vi "Read configuration.vi"(7 "force loading?":bool=TRUE, 8 "error in (no error)":errorcluster, 11 "RSA in":refnum<class "RSA.lvclass">) -> (0 "error out":errorcluster, 3 "RSA out":refnum<class "RSA.lvclass">)   [LabVIEW 2012, in "RSA.lvclass"]
doc: "Reads the XML-based configuration file and populates the configuration cluster accordingly. Configuration file name is <component ID>.xml."
uses:
  RSA.lvclass
  <vilib>/Distrio/Murmex/Murmex/Murmex.lvclass
  RSA.lvclass/RSA.ctl
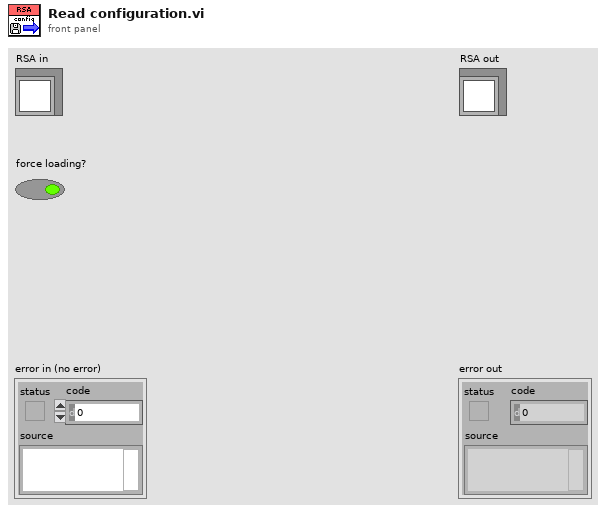
[diagram p1: front panel]
types:
  T1 = typedef "RSA.lvclass/configurationcluster.ctl" = cluster{"initialised array":dbl[]}
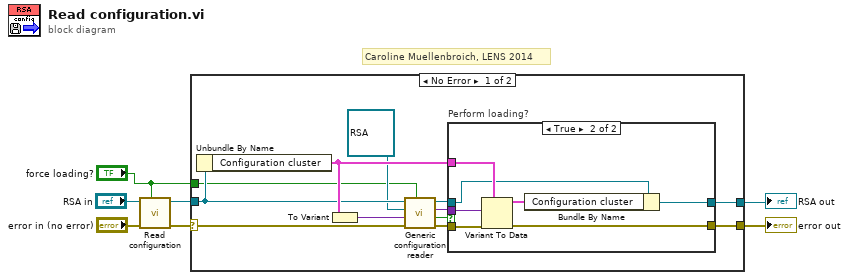
[diagram p0: block diagram]
diagram:
  # "Caroline Muellenbroich, LENS 2014"
  n1 = call-parent "Read configuration.vi"("force loading?"="force loading?", "error in (no error)"="error in (no error)", "Murmex in"="RSA in") -> ("error out"=w5:errorcluster, "Murmex out"=w4:refnum<class "RSA.lvclass">)  [unwired: 7 in]
  n2 = case shown="No Error" w5 {
    selector: w5 -> [w16 w29]
    tunnel: w4 -> [w11 w30]
    tunnel: [w18 w30] -> w3
    tunnel: [w17 w29] -> w2
    tunnel: "force loading?" -> [w8 _]
    frame No Error {
      n3 = Unbundle By Name(w11) -> ("Configuration cluster"=w19:T1)
      n4 = To Variant(anything=w19) -> (Variant=w9:variant)
      n5 = call <vilib>:"Generic configuration reader.vi"("force loading?"=w8, "error in (no error)"=w16, "configuration cluster variant"=w9, "inheritance level"=refnum<class "RSA.lvclass"> refnum ("RSA"), "Murmex in"=w11) -> ("error out"=w15:errorcluster, "loaded?"=w14:bool, "configuration data (variant)"=w13:variant, "Murmex out"=w12:refnum<class "RSA.lvclass">)  [unwired: 3 in]
      n6 = case "Perform loading?" shown="True" w14 {
        tunnel: w19 -> [_ w28]
        tunnel: [w21 w26] -> w17
        tunnel: [w20 w25] -> w18
        tunnel: w15 -> [w21 w22]
        tunnel: w12 -> [w20 w24]
        tunnel: w13 -> [_ w23]
        frame False {
        }
        frame True {
          n7 = Variant To Data(error in=w22, type=w28, Variant=w23) -> (data=w27:T1, error out=w26:errorcluster)
          n8 = Bundle By Name(cluster=w24, "Configuration cluster"=w27) -> (w25:refnum<class "RSA.lvclass">)
        }
      }
    }
    frame Error {
    }
  }
  "error out" <- w2
  "RSA out" <- w3
